vi "pPixel to Image.vi"(0 "Image in":T2, 2 "pPixel16":u16[](array[numeric]), 3 "pPixel8":u8[](array[numeric]), 5 "Error In (no error)":errorcluster, 8 "BITMAPINFOHEADER":T1) -> (14 "Image out":T2, 19 "Error Out":errorcluster)   [LabVIEW 2013, in "VRI.lvlib"]
doc: "This VI is used to convert the pPixel 1D array into the Image datatype included with the NI Vision packages."
uses:
  VRI.lvlib
  <vilib>/vision/NI_Vision_Development_Module.lvlib
  <vilib>/vision/Image Controls.llb/IMAQ Image.ctl
  _Type Defs/BITMAPINFOHEADER.ctl
panel:
  # "For instructions on the use of this VI, press Ctrl+H to display the help window and move the mouse over the icon, controls, and indicators"
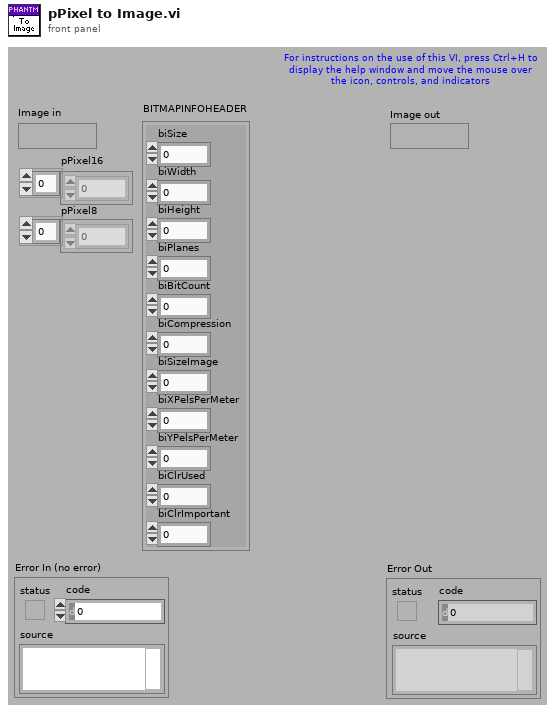
[diagram p1: front panel]
types:
  T1 = typedef "VRI.lvlib/BITMAPINFOHEADER.ctl" = cluster{"biSize":u32, "biWidth":i32, "biHeight":i32, "biPlanes":u16, "biBitCount":u16, "biCompression":u32, "biSizeImage":u32, "biXPelsPerMeter":i32, "biYPelsPerMeter":i32, "biClrUsed":u32, "biClrImportant":u32}
  T2 = typedef "IMAQ Image.ctl" = refnum<image>
  T3 = typedef "Color (U64)" = cluster{"Plane 3 (Blue)":u16, "Plane 2 (Green)":u16, "Plane 1 (Red)":u16, "Plane 4 (alpha)":u16}
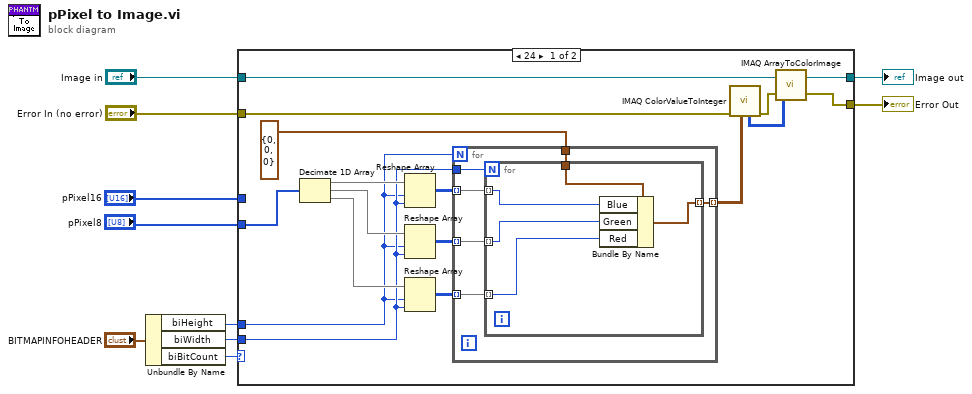
[diagram p0: block diagram]
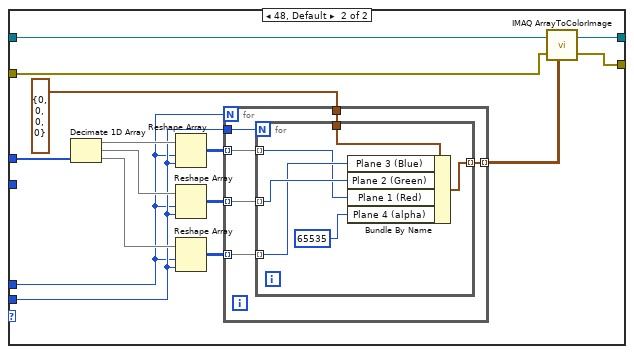
[diagram p2: hidden frame]
diagram:
  n1 = Unbundle By Name("BITMAPINFOHEADER") -> ("biHeight"=w3:i32, "biWidth"=w2:i32, "biBitCount"=w1:u16)
  n2 = case shown="24" w1 {
    tunnel: "pPixel8" -> [w19 _]
    tunnel: "pPixel16" -> [_ w45]
    tunnel: "Image in" -> [w17 w44]
    tunnel: [w18 w43] -> w7
    tunnel: [w15 w42] -> w5
    tunnel: "Error In (no error)" -> [w14 w41]
    tunnel: w2 -> [w13 w40]
    tunnel: w3 -> [w12 w39]
    frame 24 {
      n3 = Decimate 1D Array(w19) -> (w27:u8[], w26:u8[], w25:u8[])
      n4 = Reshape Array(w27, w12, w13) -> (w24:u8[][])
      n5 = Reshape Array(w26, w12, w13) -> (w23:u8[][])
      n6 = Reshape Array(w25, w12, w13) -> (w22:u8[][])
      n7 = for {
        N: w12 -> [_]
        tunnel: w13 -> [w33]
        tunnel: w24 -> [w32] mode=indexing
        tunnel: w23 -> [w31] mode=indexing
        tunnel: w22 -> [w30] mode=indexing
        tunnel: [w29] -> w21 mode=indexing
        tunnel: cluster{"Blue":u8, "Green":u8, "Red":u8} {"Blue"=0, "Green"=0, "Red"=0} ("Color (U32)") -> [w28]
        n8 = for {
          N: w33 -> [_]
          tunnel: w32 -> [w36] mode=indexing
          tunnel: w31 -> [w35] mode=indexing
          tunnel: w30 -> [w34] mode=indexing
          tunnel: [w38] -> w29 mode=indexing
          tunnel: w28 -> [w37]
          n9 = Bundle By Name(cluster=w37, "Blue"=w36, "Green"=w35, "Red"=w34) -> (w38:cluster{"Blue":u8, "Green":u8, "Red":u8})
        }
      }
      n10 = call "IMAQ ColorValueToInteger"("error in (no error)"=w14, "2D Color value array"=w21) -> ("2D U32 array"=w20:u32[][], "error out"=w16:errorcluster)  [unwired: 3 in, 2 out]
      n11 = call "IMAQ ArrayToColorImage"("Image Pixels (U32)"=w20, "Image"=w17, "error in (no error)"=w16) -> ("Image Out"=w18:T2, "error out"=w15:errorcluster)  [unwired: 1 in, 1 out]
    }
    frame 48, Default {
      n12 = Decimate 1D Array(w45) -> (w53:u16[], w52:u16[], w51:u16[])
      n13 = Reshape Array(w53, w39, w40) -> (w50:u16[][])
      n14 = Reshape Array(w52, w39, w40) -> (w49:u16[][])
      n15 = Reshape Array(w51, w39, w40) -> (w48:u16[][])
      n16 = for {
        N: w39 -> [_]
        tunnel: w40 -> [w59]
        tunnel: w50 -> [w58] mode=indexing
        tunnel: w49 -> [w57] mode=indexing
        tunnel: w48 -> [w56] mode=indexing
        tunnel: [w55] -> w47 mode=indexing
        tunnel: T3 {"Plane 3 (Blue)"=0, "Plane 2 (Green)"=0, "Plane 1 (Red)"=0, "Plane 4 (alpha)"=0} ("Color (U64)") -> [w54]
        n17 = for {
          N: w59 -> [_]
          tunnel: w58 -> [w60] mode=indexing
          tunnel: w57 -> [w63] mode=indexing
          tunnel: w56 -> [w61] mode=indexing
          tunnel: [w65] -> w55 mode=indexing
          tunnel: w54 -> [w64]
          n18 = Bundle By Name(cluster=w64, "Plane 3 (Blue)"=w61, "Plane 2 (Green)"=w63, "Plane 1 (Red)"=w60, "Plane 4 (alpha)"=u16 65535) -> (w65:T3)
        }
      }
      n19 = call "IMAQ ArrayToColorImage"("Image"=w44, "Image Pixels (U64)"=w47, "error in (no error)"=w41) -> ("Image Out"=w43:T2, "error out"=w42:errorcluster)  [unwired: 1 in, 1 out]
    }
  }
  "Image out" <- w7
  "Error Out" <- w5
